vi "3D_update (SubVI).vi"(7 "SceneGraphDisp Refnum":refnum<vi>, 9 "Altitude [m]":dbl, 10 "Euler Angles [deg]":dbl[](array[numeric]), 11 "SceneObject in":refnum<vi>) -> ()   [LabVIEW 2017]
uses:
  <vilib>/Analysis/coordinate.llb/Euler Rotation Order.ctl
  <vilib>/picture/3D Picture Control/NI_3D Picture Control.lvlib
  <vilib>/Analysis/NI_AALPro.lvlib
  <vilib>/Utility/miscctls.llb/LV3DPointTypeDef.ctl
panel:
  out "B-frame [m]":cluster{"X":sgl, "Y":sgl, "Z":sgl}
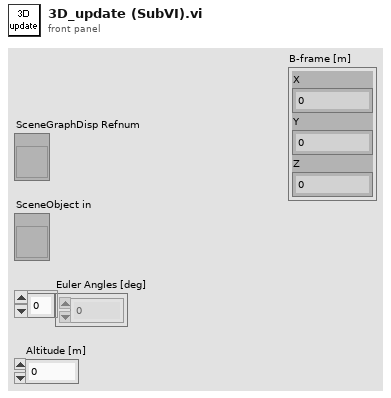
[diagram p1: front panel]
types:
  T1 = typedef "NI_AALPro.lvlib/Euler Rotation Order.ctl" = u16
  T2 = typedef "LV3DPointTypeDef.ctl" = cluster{"X":sgl, "Y":sgl, "Z":sgl}
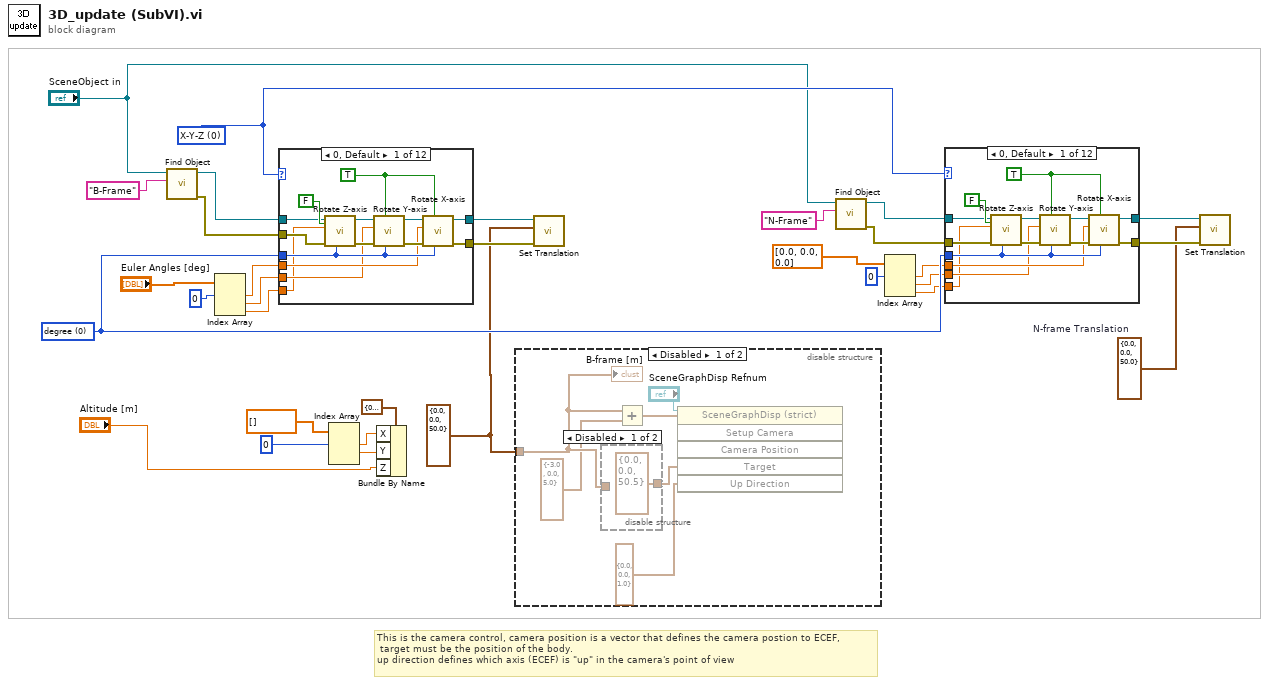
[diagram p0: block diagram]
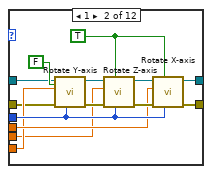
[diagram p4: hidden frame]
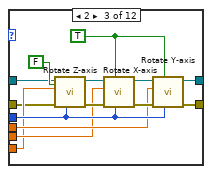
[diagram p5: hidden frame]
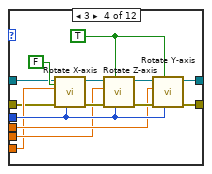
[diagram p6: hidden frame]
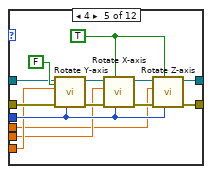
[diagram p7: hidden frame]
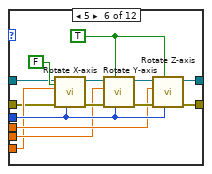
[diagram p8: hidden frame]
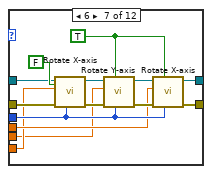
[diagram p9: hidden frame]
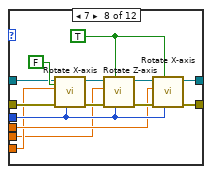
[diagram p10: hidden frame]
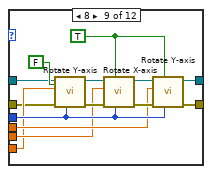
[diagram p11: hidden frame]
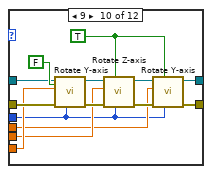
[diagram p12: hidden frame]
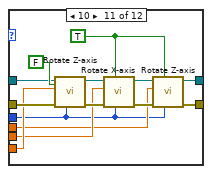
[diagram p13: hidden frame]
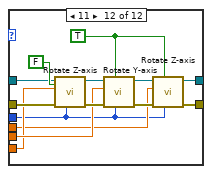
[diagram p14: hidden frame]
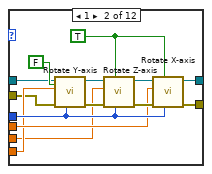
[diagram p15: hidden frame]
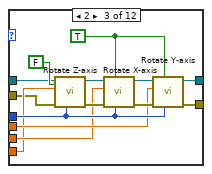
[diagram p16: hidden frame]
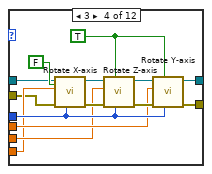
[diagram p17: hidden frame]
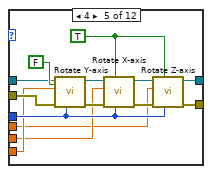
[diagram p18: hidden frame]
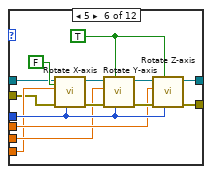
[diagram p19: hidden frame]
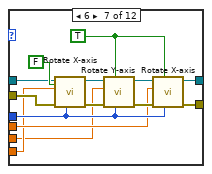
[diagram p20: hidden frame]
diagram:
  w1 = cluster{"X":sgl, "Y":sgl, "Z":sgl} {"X"=0.0, "Y"=0.0, "Z"=50.0} ("N-frame Translation")
  w22 = T1 0 items=["X-Y-Z", "X-Z-Y", "Y-X-Z", "Y-Z-X", "Z-X-Y", "Z-Y-X", "X-Y-X", "X-Z-X", "Y-X-Y", "Y-Z-Y", "Z-X-Z", "Z-Y-Z"] ("rotation order")
  w11 = cluster{"X":sgl, "Y":sgl, "Z":sgl} {"X"=0.0, "Y"=0.0, "Z"=50.0}  # N-frame Translation
  w31 = u16 0 items=["degree", "radians"] ("angle unit")
  # "This is the camera control, camera position is a vector that defines the camera postion to ECEF,\n target must be the position of the body. \nup direction defines which axis (ECEF) is \"up\" in the camera's point of view"
  n1 = call <vilib>:"Find Object.vi"("Object Name"="B-Frame", "Scene Refnum"="SceneObject in") -> ("error out"=w5:errorcluster, "Object Refnum"=w4:refnum<vi>)  [unwired: 8 in]
  n2 = Index Array(array="Euler Angles [deg]", index #1=0 ("index")) -> (element #1=w3:dbl, element #2=w6:dbl, element #3=w7:dbl)  [unwired: 2 in]
  n3 = case shown="0, Default" w22 {
    tunnel: w3 -> [w36 w52 w66 w80 w90 w108 w122 w136 w150 w161 w175 w189]
    tunnel: w4 -> [w39 w49 w62 w76 w94 w104 w121 w135 w146 w165 w179 w193]
    tunnel: w5 -> [w38 w48 w63 w77 w93 w105 w120 w134 w147 w164 w178 w192]
    tunnel: w6 -> [w35 w50 w65 w79 w91 w107 w118 w132 w149 w162 w176 w191]
    tunnel: w7 -> [w34 w51 w64 w78 w92 w106 w119 w133 w148 w163 w177 w190]
    tunnel: w31 -> [w37 w53 w67 w81 w95 w109 w123 w137 w151 w160 w174 w188]
    tunnel: [w33 w47 w61 w75 w89 w103 w117 w131 w145 w159 w173 w187] -> w9
    tunnel: [w32 w46 w60 w74 w88 w102 w116 w130 w144 w158 w172 w186] -> w10
    frame 0, Default {
      w45 = TRUE ("Relative?")
      n4 = call <vilib>:"Rotate Z-axis.vi"("angle unit"=w37, "Relative?"=FALSE, "error in (no error)"=w38, "angle"=w34, "Scene Object In"=w39) -> ("error out"=w42:errorcluster, "Scene Object Out"=w43:refnum<vi>)  [unwired: 5 in]
      n5 = call <vilib>:"Rotate Y-axis.vi"("angle unit"=w37, "Relative?"=w45, "error in (no error)"=w42, "angle"=w35, "Scene Object In"=w43) -> ("error out"=w41:errorcluster, "Scene Object Out"=w40:refnum<vi>)  [unwired: 5 in]
      n6 = call <vilib>:"Rotate X-axis.vi"("angle unit"=w37, "Relative?"=w45, "error in (no error)"=w41, "angle"=w36, "Scene Object In"=w40) -> ("error out"=w32:errorcluster, "Scene Object Out"=w33:refnum<vi>)  [unwired: 5 in]
    }
    frame 1 {
      w56 = TRUE ("Relative?")
      n7 = call <vilib>:"Rotate Y-axis.vi"("angle unit"=w53, "Relative?"=FALSE, "error in (no error)"=w48, "angle"=w51, "Scene Object In"=w49) -> ("error out"=w57:errorcluster, "Scene Object Out"=w58:refnum<vi>)  [unwired: 5 in]
      n8 = call <vilib>:"Rotate Z-axis.vi"("angle unit"=w53, "Relative?"=w56, "error in (no error)"=w57, "angle"=w50, "Scene Object In"=w58) -> ("error out"=w54:errorcluster, "Scene Object Out"=w55:refnum<vi>)  [unwired: 5 in]
      n9 = call <vilib>:"Rotate X-axis.vi"("angle unit"=w53, "Relative?"=w56, "error in (no error)"=w54, "angle"=w52, "Scene Object In"=w55) -> ("error out"=w46:errorcluster, "Scene Object Out"=w47:refnum<vi>)  [unwired: 5 in]
    }
    frame 2 {
      w68 = TRUE ("Relative?")
      n10 = call <vilib>:"Rotate Z-axis.vi"("angle unit"=w67, "Relative?"=FALSE, "error in (no error)"=w63, "angle"=w64, "Scene Object In"=w62) -> ("error out"=w71:errorcluster, "Scene Object Out"=w72:refnum<vi>)  [unwired: 5 in]
      n11 = call <vilib>:"Rotate X-axis.vi"("angle unit"=w67, "Relative?"=w68, "error in (no error)"=w71, "angle"=w65, "Scene Object In"=w72) -> ("error out"=w69:errorcluster, "Scene Object Out"=w70:refnum<vi>)  [unwired: 5 in]
      n12 = call <vilib>:"Rotate Y-axis.vi"("angle unit"=w67, "Relative?"=w68, "error in (no error)"=w69, "angle"=w66, "Scene Object In"=w70) -> ("error out"=w60:errorcluster, "Scene Object Out"=w61:refnum<vi>)  [unwired: 5 in]
    }
    frame 3 {
      w86 = TRUE ("Relative?")
      n13 = call <vilib>:"Rotate X-axis.vi"("angle unit"=w81, "Relative?"=FALSE, "error in (no error)"=w77, "angle"=w78, "Scene Object In"=w76) -> ("error out"=w84:errorcluster, "Scene Object Out"=w85:refnum<vi>)  [unwired: 5 in]
      n14 = call <vilib>:"Rotate Z-axis.vi"("angle unit"=w81, "Relative?"=w86, "error in (no error)"=w84, "angle"=w79, "Scene Object In"=w85) -> ("error out"=w82:errorcluster, "Scene Object Out"=w83:refnum<vi>)  [unwired: 5 in]
      n15 = call <vilib>:"Rotate Y-axis.vi"("angle unit"=w81, "Relative?"=w86, "error in (no error)"=w82, "angle"=w80, "Scene Object In"=w83) -> ("error out"=w74:errorcluster, "Scene Object Out"=w75:refnum<vi>)  [unwired: 5 in]
    }
    frame 4 {
      w100 = TRUE ("Relative?")
      n16 = call <vilib>:"Rotate Y-axis.vi"("angle unit"=w95, "Relative?"=FALSE, "error in (no error)"=w93, "angle"=w92, "Scene Object In"=w94) -> ("error out"=w96:errorcluster, "Scene Object Out"=w97:refnum<vi>)  [unwired: 5 in]
      n17 = call <vilib>:"Rotate X-axis.vi"("angle unit"=w95, "Relative?"=w100, "error in (no error)"=w96, "angle"=w91, "Scene Object In"=w97) -> ("error out"=w99:errorcluster, "Scene Object Out"=w98:refnum<vi>)  [unwired: 5 in]
      n18 = call <vilib>:"Rotate Z-axis.vi"("angle unit"=w95, "Relative?"=w100, "error in (no error)"=w99, "angle"=w90, "Scene Object In"=w98) -> ("error out"=w88:errorcluster, "Scene Object Out"=w89:refnum<vi>)  [unwired: 5 in]
    }
    frame 5 {
      w113 = TRUE ("Relative?")
      n19 = call <vilib>:"Rotate X-axis.vi"("angle unit"=w109, "Relative?"=FALSE, "error in (no error)"=w105, "angle"=w106, "Scene Object In"=w104) -> ("error out"=w111:errorcluster, "Scene Object Out"=w112:refnum<vi>)  [unwired: 5 in]
      n20 = call <vilib>:"Rotate Y-axis.vi"("angle unit"=w109, "Relative?"=w113, "error in (no error)"=w111, "angle"=w107, "Scene Object In"=w112) -> ("error out"=w115:errorcluster, "Scene Object Out"=w114:refnum<vi>)  [unwired: 5 in]
      n21 = call <vilib>:"Rotate Z-axis.vi"("angle unit"=w109, "Relative?"=w113, "error in (no error)"=w115, "angle"=w108, "Scene Object In"=w114) -> ("error out"=w102:errorcluster, "Scene Object Out"=w103:refnum<vi>)  [unwired: 5 in]
    }
    frame 6 {
      w126 = TRUE ("Relative?")
      n22 = call <vilib>:"Rotate X-axis.vi"("angle unit"=w123, "Relative?"=FALSE, "error in (no error)"=w120, "angle"=w119, "Scene Object In"=w121) -> ("error out"=w128:errorcluster, "Scene Object Out"=w129:refnum<vi>)  [unwired: 5 in]
      n23 = call <vilib>:"Rotate Y-axis.vi"("angle unit"=w123, "Relative?"=w126, "error in (no error)"=w128, "angle"=w118, "Scene Object In"=w129) -> ("error out"=w124:errorcluster, "Scene Object Out"=w125:refnum<vi>)  [unwired: 5 in]
      n24 = call <vilib>:"Rotate X-axis.vi"("angle unit"=w123, "Relative?"=w126, "error in (no error)"=w124, "angle"=w122, "Scene Object In"=w125) -> ("error out"=w116:errorcluster, "Scene Object Out"=w117:refnum<vi>)  [unwired: 5 in]
    }
    frame 7 {
      w142 = TRUE ("Relative?")
      n25 = call <vilib>:"Rotate X-axis.vi"("angle unit"=w137, "Relative?"=FALSE, "error in (no error)"=w134, "angle"=w133, "Scene Object In"=w135) -> ("error out"=w140:errorcluster, "Scene Object Out"=w141:refnum<vi>)  [unwired: 5 in]
      n26 = call <vilib>:"Rotate Z-axis.vi"("angle unit"=w137, "Relative?"=w142, "error in (no error)"=w140, "angle"=w132, "Scene Object In"=w141) -> ("error out"=w139:errorcluster, "Scene Object Out"=w138:refnum<vi>)  [unwired: 5 in]
      n27 = call <vilib>:"Rotate X-axis.vi"("angle unit"=w137, "Relative?"=w142, "error in (no error)"=w139, "angle"=w136, "Scene Object In"=w138) -> ("error out"=w130:errorcluster, "Scene Object Out"=w131:refnum<vi>)  [unwired: 5 in]
    }
    frame 8 {
      w156 = TRUE ("Relative?")
      n28 = call <vilib>:"Rotate Y-axis.vi"("angle unit"=w151, "Relative?"=FALSE, "error in (no error)"=w147, "angle"=w148, "Scene Object In"=w146) -> ("error out"=w154:errorcluster, "Scene Object Out"=w155:refnum<vi>)  [unwired: 5 in]
      n29 = call <vilib>:"Rotate X-axis.vi"("angle unit"=w151, "Relative?"=w156, "error in (no error)"=w154, "angle"=w149, "Scene Object In"=w155) -> ("error out"=w153:errorcluster, "Scene Object Out"=w152:refnum<vi>)  [unwired: 5 in]
      n30 = call <vilib>:"Rotate Y-axis.vi"("angle unit"=w151, "Relative?"=w156, "error in (no error)"=w153, "angle"=w150, "Scene Object In"=w152) -> ("error out"=w144:errorcluster, "Scene Object Out"=w145:refnum<vi>)  [unwired: 5 in]
    }
    frame 9 {
      w170 = TRUE ("Relative?")
      n31 = call <vilib>:"Rotate Y-axis.vi"("angle unit"=w160, "Relative?"=FALSE, "error in (no error)"=w164, "angle"=w163, "Scene Object In"=w165) -> ("error out"=w168:errorcluster, "Scene Object Out"=w169:refnum<vi>)  [unwired: 5 in]
      n32 = call <vilib>:"Rotate Z-axis.vi"("angle unit"=w160, "Relative?"=w170, "error in (no error)"=w168, "angle"=w162, "Scene Object In"=w169) -> ("error out"=w167:errorcluster, "Scene Object Out"=w166:refnum<vi>)  [unwired: 5 in]
      n33 = call <vilib>:"Rotate Y-axis.vi"("angle unit"=w160, "Relative?"=w170, "error in (no error)"=w167, "angle"=w161, "Scene Object In"=w166) -> ("error out"=w158:errorcluster, "Scene Object Out"=w159:refnum<vi>)  [unwired: 5 in]
    }
    frame 10 {
      w184 = TRUE ("Relative?")
      n34 = call <vilib>:"Rotate Z-axis.vi"("angle unit"=w174, "Relative?"=FALSE, "error in (no error)"=w178, "angle"=w177, "Scene Object In"=w179) -> ("error out"=w182:errorcluster, "Scene Object Out"=w183:refnum<vi>)  [unwired: 5 in]
      n35 = call <vilib>:"Rotate X-axis.vi"("angle unit"=w174, "Relative?"=w184, "error in (no error)"=w182, "angle"=w176, "Scene Object In"=w183) -> ("error out"=w181:errorcluster, "Scene Object Out"=w180:refnum<vi>)  [unwired: 5 in]
      n36 = call <vilib>:"Rotate Z-axis.vi"("angle unit"=w174, "Relative?"=w184, "error in (no error)"=w181, "angle"=w175, "Scene Object In"=w180) -> ("error out"=w172:errorcluster, "Scene Object Out"=w173:refnum<vi>)  [unwired: 5 in]
    }
    frame 11 {
      w198 = TRUE ("Relative?")
      n37 = call <vilib>:"Rotate Z-axis.vi"("angle unit"=w188, "Relative?"=FALSE, "error in (no error)"=w192, "angle"=w190, "Scene Object In"=w193) -> ("error out"=w196:errorcluster, "Scene Object Out"=w197:refnum<vi>)  [unwired: 5 in]
      n38 = call <vilib>:"Rotate Y-axis.vi"("angle unit"=w188, "Relative?"=w198, "error in (no error)"=w196, "angle"=w191, "Scene Object In"=w197) -> ("error out"=w195:errorcluster, "Scene Object Out"=w194:refnum<vi>)  [unwired: 5 in]
      n39 = call <vilib>:"Rotate Z-axis.vi"("angle unit"=w188, "Relative?"=w198, "error in (no error)"=w195, "angle"=w189, "Scene Object In"=w194) -> ("error out"=w186:errorcluster, "Scene Object Out"=w187:refnum<vi>)  [unwired: 5 in]
    }
  }
  n40 = Index Array(array=dbl[] [], index #1=0 ("index")) -> (element #1=w25:dbl, element #2=w26:dbl)  [unwired: 2 in, 1 out]
  n41 = Bundle By Name(cluster=cluster{"X":sgl, "Y":sgl, "Z":sgl} {"X"=0.0, "Y"=0.0, "Z"=0.0} ("B-frame Translation in"), "X"=w25, "Y"=w26, "Z"="Altitude [m]") -> ()  [unwired: 1 out]
  n42 = disable-structure shown="Disabled" {
    disable-tunnel: w1 -> [w205 _]
    frame Disabled {
      n43 = disable-structure shown="Disabled" {
        disable-tunnel: [T2 {"X"=0.0, "Y"=0.0, "Z"=50.5} ("Target") w207] -> w203
        disable-tunnel: w205 -> [_ w207]
        frame Disabled {
        }
        frame Enabled {
        }
      }
      n44 = Add(x=w205, y=T2 {"X"=-3.0, "Y"=0.0, "Z"=5.0} ("Camera Position control")) -> (x+y=w204:T2)
      n45 = invoke on="Invoke Node" class="SceneGraphDisp (strict)" method="Setup Camera"(reference="SceneGraphDisp Refnum", "Camera Position"=w204, "Target"=w203, "Up Direction"=T2 {"X"=0.0, "Y"=0.0, "Z"=1.0}) -> ()  [unwired: 2 in, 6 out]
      "B-frame [m]" <- w205
    }
    frame Enabled {
    }
  }
  n46 = call <vilib>:"Set Translation.vi"("error in (no error)"=w10, "Translation"=w1, "Scene Object"=w9) -> ()  [unwired: 7 in, 2 out]
  n47 = call <vilib>:"Find Object.vi"("Object Name"="N-Frame", "Scene Refnum"="SceneObject in") -> ("error out"=w17:errorcluster, "Object Refnum"=w18:refnum<vi>)  [unwired: 8 in]
  n48 = Index Array(array=dbl[] [0.0, 0.0, 0.0] ("N-frame rot"), index #1=0 ("index")) -> (element #1=w19:dbl, element #2=w16:dbl, element #3=w15:dbl)  [unwired: 2 in]
  n49 = case shown="0, Default" w22 {
    tunnel: w19 -> [w212 w228 w242 w256 w266 w284 w298 w312 w326 w337 w351 w365]
    tunnel: w18 -> [w215 w225 w238 w252 w270 w280 w297 w311 w322 w341 w355 w369]
    tunnel: w17 -> [w214 w224 w239 w253 w269 w281 w296 w310 w323 w340 w354 w368]
    tunnel: w16 -> [w211 w226 w241 w255 w267 w283 w294 w308 w325 w338 w352 w367]
    tunnel: w15 -> [w210 w227 w240 w254 w268 w282 w295 w309 w324 w339 w353 w366]
    tunnel: w31 -> [w213 w229 w243 w257 w271 w285 w299 w313 w327 w336 w350 w364]
    tunnel: [w209 w223 w237 w251 w265 w279 w293 w307 w321 w335 w349 w363] -> w13
    tunnel: [w208 w222 w236 w250 w264 w278 w292 w306 w320 w334 w348 w362] -> w12
    frame 0, Default {
      w221 = TRUE ("Relative?")
      n50 = call <vilib>:"Rotate Z-axis.vi"("angle unit"=w213, "Relative?"=FALSE, "error in (no error)"=w214, "angle"=w210, "Scene Object In"=w215) -> ("error out"=w218:errorcluster, "Scene Object Out"=w219:refnum<vi>)  [unwired: 5 in]
      n51 = call <vilib>:"Rotate Y-axis.vi"("angle unit"=w213, "Relative?"=w221, "error in (no error)"=w218, "angle"=w211, "Scene Object In"=w219) -> ("error out"=w217:errorcluster, "Scene Object Out"=w216:refnum<vi>)  [unwired: 5 in]
      n52 = call <vilib>:"Rotate X-axis.vi"("angle unit"=w213, "Relative?"=w221, "error in (no error)"=w217, "angle"=w212, "Scene Object In"=w216) -> ("error out"=w208:errorcluster, "Scene Object Out"=w209:refnum<vi>)  [unwired: 5 in]
    }
    frame 1 {
      w232 = TRUE ("Relative?")
      n53 = call <vilib>:"Rotate Y-axis.vi"("angle unit"=w229, "Relative?"=FALSE, "error in (no error)"=w224, "angle"=w227, "Scene Object In"=w225) -> ("error out"=w233:errorcluster, "Scene Object Out"=w234:refnum<vi>)  [unwired: 5 in]
      n54 = call <vilib>:"Rotate Z-axis.vi"("angle unit"=w229, "Relative?"=w232, "error in (no error)"=w233, "angle"=w226, "Scene Object In"=w234) -> ("error out"=w230:errorcluster, "Scene Object Out"=w231:refnum<vi>)  [unwired: 5 in]
      n55 = call <vilib>:"Rotate X-axis.vi"("angle unit"=w229, "Relative?"=w232, "error in (no error)"=w230, "angle"=w228, "Scene Object In"=w231) -> ("error out"=w222:errorcluster, "Scene Object Out"=w223:refnum<vi>)  [unwired: 5 in]
    }
    frame 2 {
      w244 = TRUE ("Relative?")
      n56 = call <vilib>:"Rotate Z-axis.vi"("angle unit"=w243, "Relative?"=FALSE, "error in (no error)"=w239, "angle"=w240, "Scene Object In"=w238) -> ("error out"=w247:errorcluster, "Scene Object Out"=w248:refnum<vi>)  [unwired: 5 in]
      n57 = call <vilib>:"Rotate X-axis.vi"("angle unit"=w243, "Relative?"=w244, "error in (no error)"=w247, "angle"=w241, "Scene Object In"=w248) -> ("error out"=w245:errorcluster, "Scene Object Out"=w246:refnum<vi>)  [unwired: 5 in]
      n58 = call <vilib>:"Rotate Y-axis.vi"("angle unit"=w243, "Relative?"=w244, "error in (no error)"=w245, "angle"=w242, "Scene Object In"=w246) -> ("error out"=w236:errorcluster, "Scene Object Out"=w237:refnum<vi>)  [unwired: 5 in]
    }
    frame 3 {
      w262 = TRUE ("Relative?")
      n59 = call <vilib>:"Rotate X-axis.vi"("angle unit"=w257, "Relative?"=FALSE, "error in (no error)"=w253, "angle"=w254, "Scene Object In"=w252) -> ("error out"=w260:errorcluster, "Scene Object Out"=w261:refnum<vi>)  [unwired: 5 in]
      n60 = call <vilib>:"Rotate Z-axis.vi"("angle unit"=w257, "Relative?"=w262, "error in (no error)"=w260, "angle"=w255, "Scene Object In"=w261) -> ("error out"=w258:errorcluster, "Scene Object Out"=w259:refnum<vi>)  [unwired: 5 in]
      n61 = call <vilib>:"Rotate Y-axis.vi"("angle unit"=w257, "Relative?"=w262, "error in (no error)"=w258, "angle"=w256, "Scene Object In"=w259) -> ("error out"=w250:errorcluster, "Scene Object Out"=w251:refnum<vi>)  [unwired: 5 in]
    }
    frame 4 {
      w276 = TRUE ("Relative?")
      n62 = call <vilib>:"Rotate Y-axis.vi"("angle unit"=w271, "Relative?"=FALSE, "error in (no error)"=w269, "angle"=w268, "Scene Object In"=w270) -> ("error out"=w272:errorcluster, "Scene Object Out"=w273:refnum<vi>)  [unwired: 5 in]
      n63 = call <vilib>:"Rotate X-axis.vi"("angle unit"=w271, "Relative?"=w276, "error in (no error)"=w272, "angle"=w267, "Scene Object In"=w273) -> ("error out"=w275:errorcluster, "Scene Object Out"=w274:refnum<vi>)  [unwired: 5 in]
      n64 = call <vilib>:"Rotate Z-axis.vi"("angle unit"=w271, "Relative?"=w276, "error in (no error)"=w275, "angle"=w266, "Scene Object In"=w274) -> ("error out"=w264:errorcluster, "Scene Object Out"=w265:refnum<vi>)  [unwired: 5 in]
    }
    frame 5 {
      w289 = TRUE ("Relative?")
      n65 = call <vilib>:"Rotate X-axis.vi"("angle unit"=w285, "Relative?"=FALSE, "error in (no error)"=w281, "angle"=w282, "Scene Object In"=w280) -> ("error out"=w287:errorcluster, "Scene Object Out"=w288:refnum<vi>)  [unwired: 5 in]
      n66 = call <vilib>:"Rotate Y-axis.vi"("angle unit"=w285, "Relative?"=w289, "error in (no error)"=w287, "angle"=w283, "Scene Object In"=w288) -> ("error out"=w291:errorcluster, "Scene Object Out"=w290:refnum<vi>)  [unwired: 5 in]
      n67 = call <vilib>:"Rotate Z-axis.vi"("angle unit"=w285, "Relative?"=w289, "error in (no error)"=w291, "angle"=w284, "Scene Object In"=w290) -> ("error out"=w278:errorcluster, "Scene Object Out"=w279:refnum<vi>)  [unwired: 5 in]
    }
    frame 6 {
      w302 = TRUE ("Relative?")
      n68 = call <vilib>:"Rotate X-axis.vi"("angle unit"=w299, "Relative?"=FALSE, "error in (no error)"=w296, "angle"=w295, "Scene Object In"=w297) -> ("error out"=w304:errorcluster, "Scene Object Out"=w305:refnum<vi>)  [unwired: 5 in]
      n69 = call <vilib>:"Rotate Y-axis.vi"("angle unit"=w299, "Relative?"=w302, "error in (no error)"=w304, "angle"=w294, "Scene Object In"=w305) -> ("error out"=w300:errorcluster, "Scene Object Out"=w301:refnum<vi>)  [unwired: 5 in]
      n70 = call <vilib>:"Rotate X-axis.vi"("angle unit"=w299, "Relative?"=w302, "error in (no error)"=w300, "angle"=w298, "Scene Object In"=w301) -> ("error out"=w292:errorcluster, "Scene Object Out"=w293:refnum<vi>)  [unwired: 5 in]
    }
    frame 7 {
      w318 = TRUE ("Relative?")
      n71 = call <vilib>:"Rotate X-axis.vi"("angle unit"=w313, "Relative?"=FALSE, "error in (no error)"=w310, "angle"=w309, "Scene Object In"=w311) -> ("error out"=w316:errorcluster, "Scene Object Out"=w317:refnum<vi>)  [unwired: 5 in]
      n72 = call <vilib>:"Rotate Z-axis.vi"("angle unit"=w313, "Relative?"=w318, "error in (no error)"=w316, "angle"=w308, "Scene Object In"=w317) -> ("error out"=w315:errorcluster, "Scene Object Out"=w314:refnum<vi>)  [unwired: 5 in]
      n73 = call <vilib>:"Rotate X-axis.vi"("angle unit"=w313, "Relative?"=w318, "error in (no error)"=w315, "angle"=w312, "Scene Object In"=w314) -> ("error out"=w306:errorcluster, "Scene Object Out"=w307:refnum<vi>)  [unwired: 5 in]
    }
    frame 8 {
      w332 = TRUE ("Relative?")
      n74 = call <vilib>:"Rotate Y-axis.vi"("angle unit"=w327, "Relative?"=FALSE, "error in (no error)"=w323, "angle"=w324, "Scene Object In"=w322) -> ("error out"=w330:errorcluster, "Scene Object Out"=w331:refnum<vi>)  [unwired: 5 in]
      n75 = call <vilib>:"Rotate X-axis.vi"("angle unit"=w327, "Relative?"=w332, "error in (no error)"=w330, "angle"=w325, "Scene Object In"=w331) -> ("error out"=w329:errorcluster, "Scene Object Out"=w328:refnum<vi>)  [unwired: 5 in]
      n76 = call <vilib>:"Rotate Y-axis.vi"("angle unit"=w327, "Relative?"=w332, "error in (no error)"=w329, "angle"=w326, "Scene Object In"=w328) -> ("error out"=w320:errorcluster, "Scene Object Out"=w321:refnum<vi>)  [unwired: 5 in]
    }
    frame 9 {
      w346 = TRUE ("Relative?")
      n77 = call <vilib>:"Rotate Y-axis.vi"("angle unit"=w336, "Relative?"=FALSE, "error in (no error)"=w340, "angle"=w339, "Scene Object In"=w341) -> ("error out"=w344:errorcluster, "Scene Object Out"=w345:refnum<vi>)  [unwired: 5 in]
      n78 = call <vilib>:"Rotate Z-axis.vi"("angle unit"=w336, "Relative?"=w346, "error in (no error)"=w344, "angle"=w338, "Scene Object In"=w345) -> ("error out"=w343:errorcluster, "Scene Object Out"=w342:refnum<vi>)  [unwired: 5 in]
      n79 = call <vilib>:"Rotate Y-axis.vi"("angle unit"=w336, "Relative?"=w346, "error in (no error)"=w343, "angle"=w337, "Scene Object In"=w342) -> ("error out"=w334:errorcluster, "Scene Object Out"=w335:refnum<vi>)  [unwired: 5 in]
    }
    frame 10 {
      w360 = TRUE ("Relative?")
      n80 = call <vilib>:"Rotate Z-axis.vi"("angle unit"=w350, "Relative?"=FALSE, "error in (no error)"=w354, "angle"=w353, "Scene Object In"=w355) -> ("error out"=w358:errorcluster, "Scene Object Out"=w359:refnum<vi>)  [unwired: 5 in]
      n81 = call <vilib>:"Rotate X-axis.vi"("angle unit"=w350, "Relative?"=w360, "error in (no error)"=w358, "angle"=w352, "Scene Object In"=w359) -> ("error out"=w357:errorcluster, "Scene Object Out"=w356:refnum<vi>)  [unwired: 5 in]
      n82 = call <vilib>:"Rotate Z-axis.vi"("angle unit"=w350, "Relative?"=w360, "error in (no error)"=w357, "angle"=w351, "Scene Object In"=w356) -> ("error out"=w348:errorcluster, "Scene Object Out"=w349:refnum<vi>)  [unwired: 5 in]
    }
    frame 11 {
      w374 = TRUE ("Relative?")
      n83 = call <vilib>:"Rotate Z-axis.vi"("angle unit"=w364, "Relative?"=FALSE, "error in (no error)"=w368, "angle"=w366, "Scene Object In"=w369) -> ("error out"=w372:errorcluster, "Scene Object Out"=w373:refnum<vi>)  [unwired: 5 in]
      n84 = call <vilib>:"Rotate Y-axis.vi"("angle unit"=w364, "Relative?"=w374, "error in (no error)"=w372, "angle"=w367, "Scene Object In"=w373) -> ("error out"=w371:errorcluster, "Scene Object Out"=w370:refnum<vi>)  [unwired: 5 in]
      n85 = call <vilib>:"Rotate Z-axis.vi"("angle unit"=w364, "Relative?"=w374, "error in (no error)"=w371, "angle"=w365, "Scene Object In"=w370) -> ("error out"=w362:errorcluster, "Scene Object Out"=w363:refnum<vi>)  [unwired: 5 in]
    }
  }
  n86 = call <vilib>:"Set Translation.vi"("error in (no error)"=w12, "Translation"=w11, "Scene Object"=w13) -> ()  [unwired: 7 in, 2 out]
